vi "fibonacci.vi"() -> ()   [LabVIEW 2023]
panel:
  out "Array":dbl[](array[numeric])
  in  "Numeric":dbl
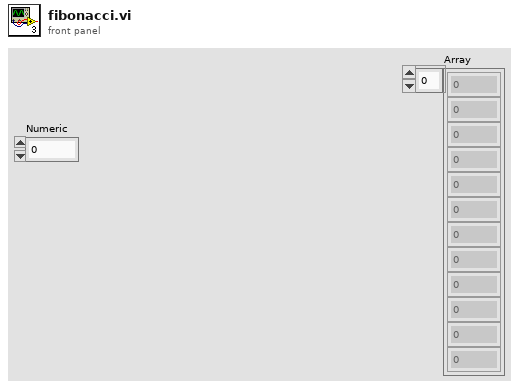
[diagram p1: front panel]
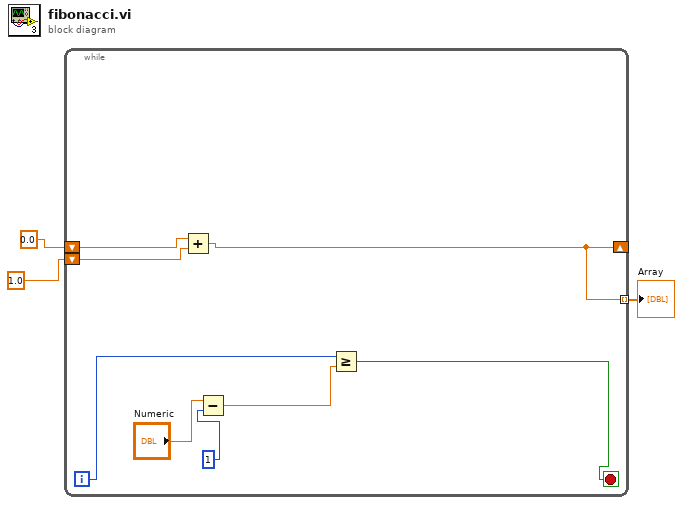
[diagram p0: block diagram]
diagram:
  n1 = while {
    shift-right: [w9] -> _
    shift-left: 0.0 -> [w11]
    shift-left: 1.0 -> [w10]
    tunnel: [w9] -> w1 mode=indexing
    i -> [w6]
    stop <- w7 stop-if-true
    n2 = Add(x=w11, y=w10) -> (x+y=w9:dbl)
    n3 = Subtract(x="Numeric", y=1) -> (x-y=w8:dbl)
    n4 = Greater Or Equal?(x=w6, y=w8) -> (x >= y?=w7:bool)
  }
  "Array" <- w1
